vi "Reset.vi"(8 "Error In":errorcluster, 11 "Keithley 7001 In":refnum<visa-resource-name>) -> (0 "Error Out":errorcluster, 3 "Keithley 7001 Out":refnum<visa-resource-name>)   [LabVIEW 2012, in "Keithley-7001.lvlib"]
uses:
  Keithley-7001.lvlib
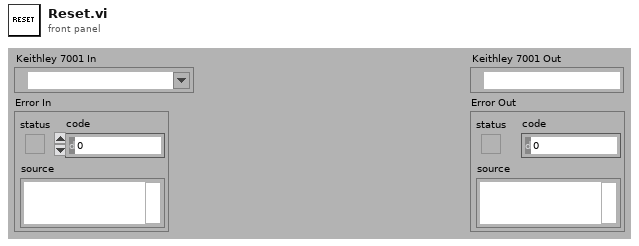
[diagram p1: front panel]
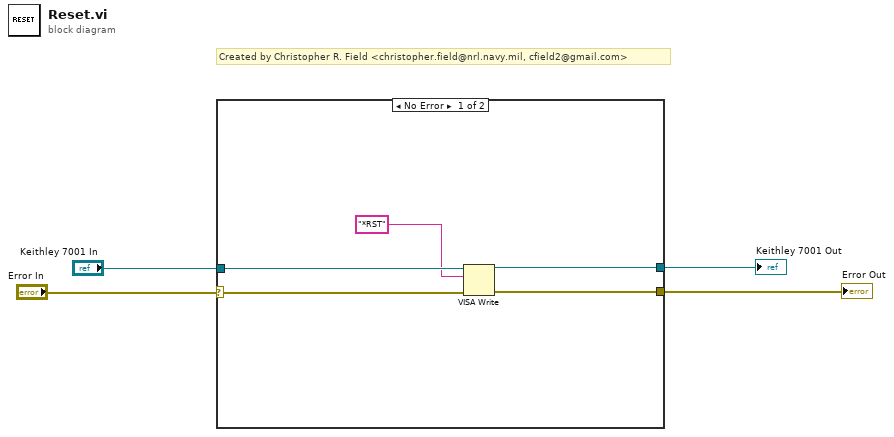
[diagram p0: block diagram]
diagram:
  # "Created by Christopher R. Field <christopher.field@nrl.navy.mil, cfield2@gmail.com>"
  n1 = case shown="No Error" "Error In" {
    selector: "Error In" -> [w5 w11]
    tunnel: "Keithley 7001 In" -> [w9 w10]
    tunnel: [w8 w10] -> w3
    tunnel: [w7 w11] -> w2
    frame No Error {
      n2 = VISA Write(VISA resource name=w9, write buffer="*RST", error in (no error)=w5) -> (VISA resource name out=w8:refnum<visa-resource-name>, error out=w7:errorcluster)  [unwired: 1 out]
    }
    frame Error {
    }
  }
  "Keithley 7001 Out" <- w3
  "Error Out" <- w2
